vi "functional global counter 1.vi"() -> ()   [LabVIEW 2010]
uses:
  Functional Global Command.ctl
panel:
  out "카운트 1":i32
  out "진행 중 합계":i32
  in  "정지":bool
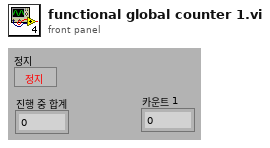
[diagram p1: front panel]
types:
  T1 = typedef "Functional Global Command.ctl" = enum16{"리셋", "증가", "카운트 가져오기"}
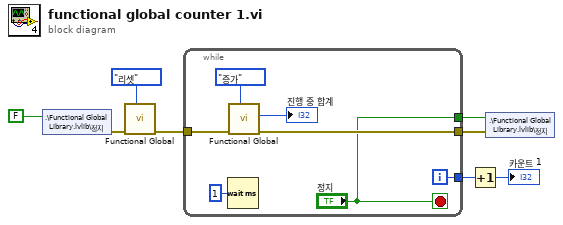
[diagram p0: block diagram]
diagram:
  n1 = shared-variable ".\\Functional Global Library.lvlib\\정지"(FALSE ("stop")) -> (error out=w2:errorcluster)  [unwired: 1 in]
  n2 = call "Functional Global.vi"("명령"=Functional_Global_Command."리셋" ("Command"), "에러 입력 (에러 없음)"=w2) -> ("에러 출력"=w5:errorcluster)  [unwired: 8 in, 1 out]
  n3 = while {
    tunnel: [w15] -> w8
    tunnel: [w10] -> w4
    tunnel: w5 -> [w12]
    tunnel: ["정지"] -> w3
    i -> [w15]
    stop <- "정지" stop-if-true
    n4 = Wait (ms)(milliseconds to wait=u32 1) -> ()  [unwired: 1 out]
    n5 = call "Functional Global.vi"("명령"=Functional_Global_Command."증가" ("Command"), "에러 입력 (에러 없음)"=w12) -> ("에러 출력"=w10:errorcluster, "카운트"=→"진행 중 합계":i32)  [unwired: 8 in]
  }
  n6 = Increment(x=w8) -> (x+1=→"카운트 1":i32)
  n7 = shared-variable ".\\Functional Global Library.lvlib\\정지"(w3, error in=w4) -> ()  [unwired: 1 out]
